vi "VsItemMap.vi"(7 "action (Set)":enum16{"Set", "Get"}(ring), 9 "Variant":variant, 10 "name":string) -> (1 "Variant out":variant)   [LabVIEW 2020]
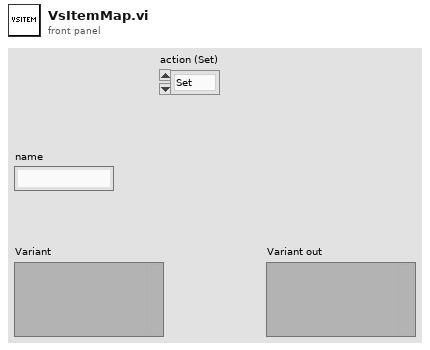
[diagram p1: front panel]
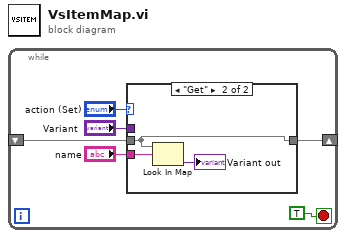
[diagram p0: block diagram]
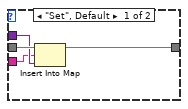
[diagram p2: hidden frame]
diagram:
  n1 = while {
    shift-right: [w6] -> _
    shift-left: _ -> [w3]
    stop <- TRUE stop-if-true
    n2 = case shown="\"Get\"" "action (Set)" {
      tunnel: [w9 w13] -> w6
      tunnel: w3 -> [w10 w13]
      tunnel: "Variant" -> [w8 _]
      tunnel: "name" -> [w7 w12]
      frame "Set", Default {
        n3 = Insert Into Map(map in=w10, key=w7, value=w8) -> (map out=w9:map{string, variant})  [unwired: 2 out]
      }
      frame "Get" {
        n4 = Look In Map(map=w13, key=w12) -> (value=→"Variant out":variant)  [unwired: 1 in, 1 out]
      }
    }
  }
